vi "AD7714 4CH Initialize.vi"(11 "I/O Cluster In":T1) -> (3 "I/O Cluster Out":T1)   [LabVIEW 2016, in "jmslib.lvlib"]
uses:
  jmslib.lvlib
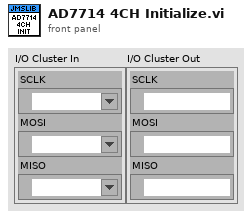
[diagram p1: front panel]
types:
  T1 = cluster{"SCLK":refnum<k21>, "MOSI":refnum<k21>, "MISO":refnum<k21>}
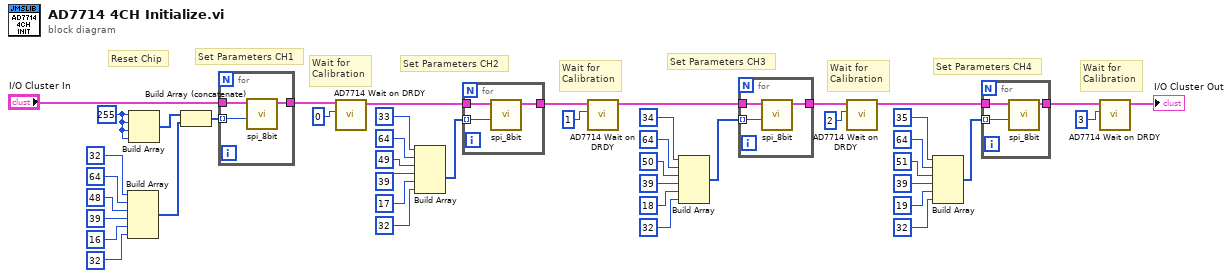
[diagram p0: block diagram]
diagram:
  w44 = 255 ("number")
  # "Wait for\nCalibration"
  # "Set Parameters CH4"
  # "Wait for\nCalibration"
  # "Set Parameters CH3"
  # "Wait for\nCalibration"
  # "Set Parameters CH2"
  # "Wait for\nCalibration"
  # "Set Parameters CH1"
  # "Reset Chip"
  n1 = Build Array(32 ("number"), 64 ("number"), 48 ("number"), 39 ("number"), 16 ("number"), 32 ("number")) -> (w36:i32[])
  n2 = Build Array(w44, w44, w44, w44) -> (w37:i32[])
  n3 = Build Array (concatenate)(w37, w36) -> (w35:i32[])
  n4 = for {
    tunnel: w35 -> [w46] mode=indexing
    tunnel: "I/O Cluster In" -> [w47]
    tunnel: [w45] -> w13
    n5 = call "spi_8bit.vi"("Hex"=w46, "I/O Cluster In"=w47) -> ("I/O Cluster Out"=w45:T1)  [unwired: 9 in]
  }
  n6 = call "AD7714 Wait on DRDY.vi"("Channel"=i16 0, "I/O Cluster In"=w13) -> ("I/O Cluster Out"=w11:T1)  [unwired: 7 in, 2 out]
  n7 = Build Array(33 ("number"), 64 ("number"), 49 ("number"), 39 ("number"), 17 ("number"), 32 ("number")) -> (w28:i32[])
  n8 = for {
    tunnel: w28 -> [w50] mode=indexing
    tunnel: w11 -> [w49]
    tunnel: [w48] -> w9
    n9 = call "spi_8bit.vi"("Hex"=w50, "I/O Cluster In"=w49) -> ("I/O Cluster Out"=w48:T1)  [unwired: 9 in]
  }
  n10 = call "AD7714 Wait on DRDY.vi"("Channel"=i16 1, "I/O Cluster In"=w9) -> ("I/O Cluster Out"=w8:T1)  [unwired: 7 in, 2 out]
  n11 = Build Array(34 ("number"), 64 ("number"), 50 ("number"), 39 ("number"), 18 ("number"), 32 ("number")) -> (w21:i32[])
  n12 = for {
    tunnel: w21 -> [w53] mode=indexing
    tunnel: w8 -> [w52]
    tunnel: [w51] -> w6
    n13 = call "spi_8bit.vi"("Hex"=w53, "I/O Cluster In"=w52) -> ("I/O Cluster Out"=w51:T1)  [unwired: 9 in]
  }
  n14 = call "AD7714 Wait on DRDY.vi"("Channel"=i16 2, "I/O Cluster In"=w6) -> ("I/O Cluster Out"=w4:T1)  [unwired: 7 in, 2 out]
  n15 = Build Array(35 ("number"), 64 ("number"), 51 ("number"), 39 ("number"), 19 ("number"), 32 ("number")) -> (w5:i32[])
  n16 = for {
    tunnel: w5 -> [w56] mode=indexing
    tunnel: w4 -> [w55]
    tunnel: [w54] -> w2
    n17 = call "spi_8bit.vi"("Hex"=w56, "I/O Cluster In"=w55) -> ("I/O Cluster Out"=w54:T1)  [unwired: 9 in]
  }
  n18 = call "AD7714 Wait on DRDY.vi"("Channel"=i16 3, "I/O Cluster In"=w2) -> ("I/O Cluster Out"=→"I/O Cluster Out":T1)  [unwired: 7 in, 2 out]
